vi "Destroy.vi"(8 "error in (no error)":errorcluster, 11 "reference in":refnum<class "FileDataSource.lvclass">) -> (0 "error out":errorcluster, 3 "reference out":refnum<class "FileDataSource.lvclass">)   [LabVIEW 2020, in "FileDataSource.lvclass"]
uses:
  FileDataSource.lvclass
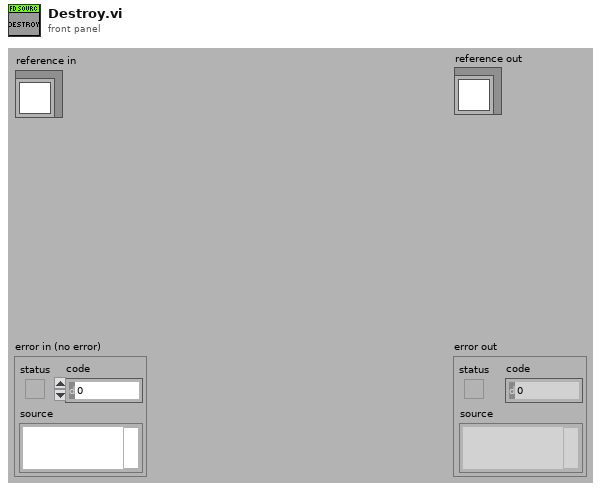
[diagram p1: front panel]
types:
  T1 = typedef "FileDataSource.lvclass/ObjectAttributes.ctl" = cluster{"Name":string}
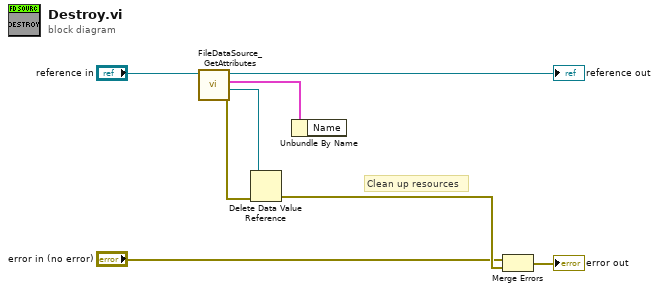
[diagram p0: block diagram]
diagram:
  # "Clean up resources"
  n1 = call "FileDataSource_GetAttributes.vi"("reference in"="reference in") -> ("error out"=w5:errorcluster, "DataRef"=w4:refnum<data-value>, "Data"=w3:T1, "reference out"=→"reference out":refnum<class "FileDataSource.lvclass">)  [unwired: 7 in]
  n2 = Delete Data Value Reference(data value reference=w4, error in=w5) -> (error out=w2:errorcluster)  [unwired: 1 out]
  n3 = Unbundle By Name(w3) -> ()  [unwired: 1 out]
  n4 = Merge Errors("error in (no error)", w2) -> (→"error out":errorcluster)
